vi "ConsolidateTerminals.vi"(1 "Terminal Set":T1(array[cluster])) -> (0 "Terminal Set":T1(array[cluster]))   [LabVIEW 2012, in "CThread.lvlib"]
uses:
  CThread.lvlib
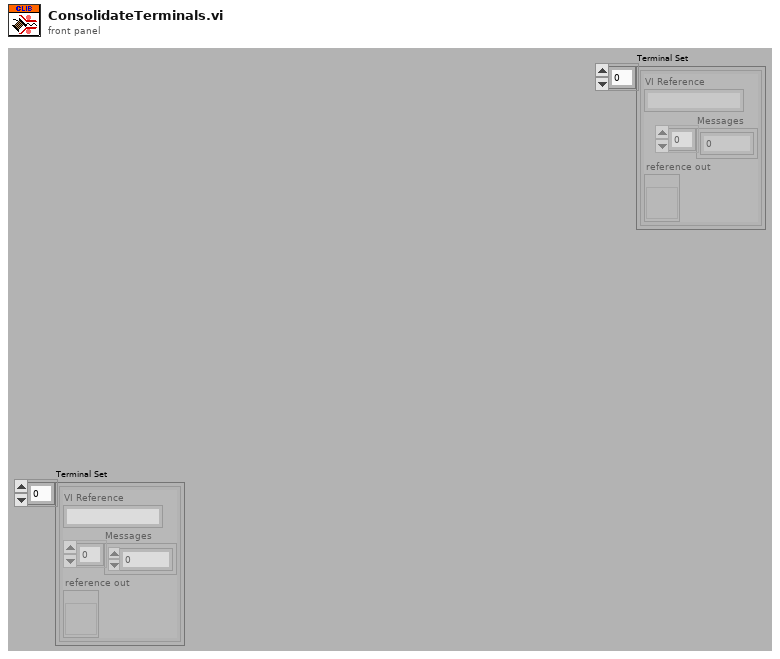
[diagram p1: front panel]
types:
  T1 = cluster{"VI Reference":string, "Messages":u8[], "reference out":refnum<vi>}[]
  T2 = cluster{"VI Reference":string, "Messages":u8[], "reference out":refnum<vi>}
  T3 = cluster{"VI Reference":string, "Combined Messages":u8[], "reference out":refnum<vi>}
  T4 = typedef "CRef.lvlib/Master Types.ctl" = enum8{"Null", "Boolean", "U8", "I8", "U16", "I16", "U32", "I32", "U64", "I64", "Single", "Double", "Extended", "CSG", "CDB", "CXT", "Boolean(Def)", "U8(Def)", "I8(Def)", "U16(Def)", "I16(Def)", "U32(Def)", "I32(Def)", "Reserved Def", "Reserved Def1", "Single(Def)", "Double(Def)", "Reserved Def2", "Reserved Def3", "Reserved Def4", "Reserved Def5", "Unsigned(Def)", "Signed(Def)", "Real(Def)", "Reserved Def6", "Numeric(Def)", "String"}
  T5 = typedef "LVRectTypeDef.ctl" = cluster{"Left":i16, "Top":i16, "Right":i16, "Bottom":i16}
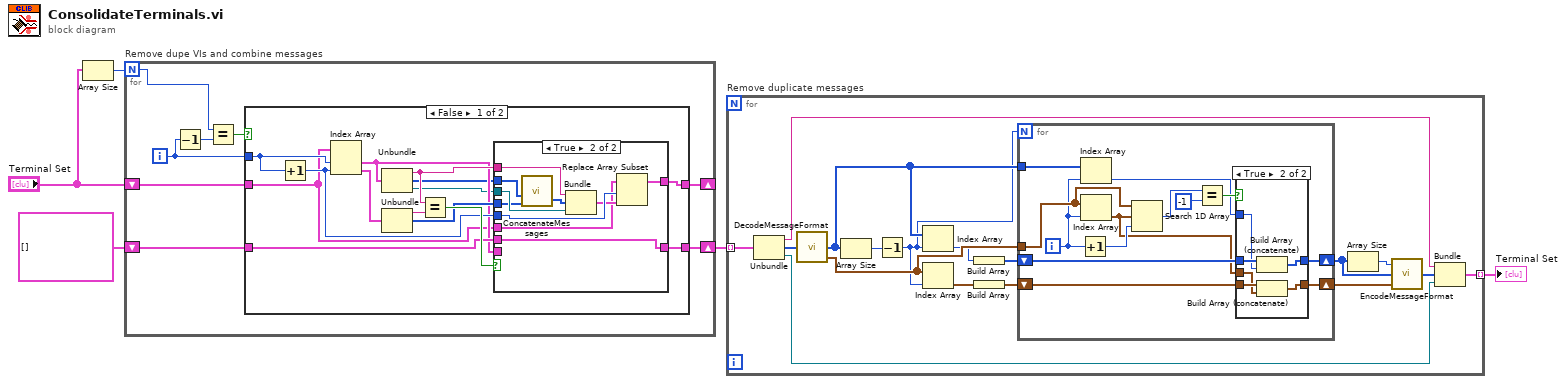
[diagram p0: block diagram]
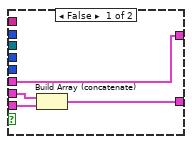
[diagram p3: hidden frame]
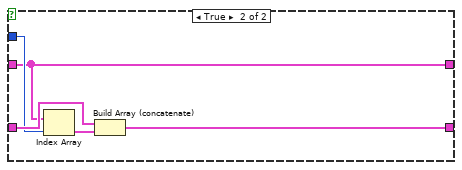
[diagram p4: hidden frame]
diagram:
  n1 = Array Size(array="Terminal Set") -> (size(s)=w5:i32)
  n2 = for "Remove dupe VIs and combine messages" {
    N: w5 -> [w13]
    shift-right: [w9] -> w2
    shift-left: T1 [] -> [w7]
    shift-right: [w6] -> _
    shift-left: "Terminal Set" -> [w8]
    i -> [w11]
    n3 = Decrement(x=w11) -> (x-1=w12:i32)
    n4 = Equal?(x=w13, y=w12) -> (x = y?=w10:bool)
    n5 = case shown="False" w10 {
      tunnel: w11 -> [w27 w44]
      tunnel: [w23 w46] -> w9
      tunnel: w8 -> [w17 w42]
      tunnel: w7 -> [w22 w45]
      tunnel: [w16 w42] -> w6
      frame False {
        n6 = Increment(x=w27) -> (x+1=w24:i32)
        n7 = Index Array(array=w17, index #1=w27, index #2=w24) -> (element #1=w18:T2, element #2=w26:T2)
        n8 = Unbundle(w18) -> ("VI Reference"=w19:string, "Messages"=w15:u8[], "reference out"=w14:refnum<vi>)
        n9 = Unbundle(w26) -> ("VI Reference"=w21:string, "Messages"=w20:u8[])  [unwired: 1 out]
        n10 = Equal?(x=w19, y=w21) -> (x = y?=w25:bool)
        n11 = case shown="True" w25 {
          tunnel: w24 -> [_ w41]
          tunnel: w22 -> [w31 w36]
          tunnel: [w30 w36] -> w23
          tunnel: w15 -> [_ w33]
          tunnel: w20 -> [_ w32]
          tunnel: w19 -> [_ w40]
          tunnel: w18 -> [w29 _]
          tunnel: w17 -> [w28 w38]
          tunnel: [w28 w37] -> w16
          tunnel: w14 -> [_ w35]
          frame False {
            n12 = Build Array (concatenate)(w31, w29) -> (w30:T1)
          }
          frame True {
            n13 = call "ConcatenateMessages.vi"("Messages 2"=w32, "Messages"=w33) -> ("Combined Messages"=w34:u8[])  [unwired: 3 in]
            n14 = Bundle("VI Reference"=w40, "Combined Messages"=w34, "reference out"=w35) -> (w39:T3)  [unwired: 1 in]
            n15 = Replace Array Subset(array=w38, new element=w39, index=w41) -> (w37:T1)
          }
        }
      }
      frame True {
        n16 = Index Array(array=w42, index=w44) -> (element=w43:T2)
        n17 = Build Array (concatenate)(w45, w43) -> (w46:T1)
      }
    }
  }
  n18 = for "Remove duplicate messages" {
    tunnel: w2 -> [w63] mode=indexing
    tunnel: [w57] -> w1 mode=indexing
    n19 = Unbundle(w63) -> ("VI Reference"=w60:string, "Messages"=w62:u8[], "reference out"=w59:refnum<vi>)
    n20 = call "DecodeMessageFormat.vi"("Messages"=w62) -> ("CRef Types"=w53:T4[], "Terminal Bounds[]"=w52:T5[])  [unwired: 2 in, 1 out]
    n21 = Array Size(array=w53) -> (size(s)=w56:i32)
    n22 = Decrement(x=w56) -> (x-1=w51:i32)
    n23 = Index Array(array=w53, index=w51) -> (element=w50:T4)
    n24 = Index Array(array=w52, index=w51) -> (element=w49:T5)
    n25 = Build Array(w50) -> (w47:T4[])
    n26 = Build Array(w49) -> (w48:T5[])
    n27 = for {
      N: w51 -> [_]
      tunnel: w53 -> [w65]
      tunnel: w52 -> [w76]
      shift-right: [w71] -> w55
      shift-left: w47 -> [w69]
      shift-right: [w70] -> w54
      shift-left: w48 -> [w68]
      i -> [w66]
      n28 = Increment(x=w66) -> (x+1=w73:i32)
      n29 = Index Array(array=w65, index=w66) -> (element=w64:T4)
      n30 = Index Array(array=w76, index=w66) -> (element=w67:T5)
      n31 = Search 1D Array(1D array=w76, element=w67, start index (0)=w73) -> (index of element=w75:i32)
      n32 = Equal?(x=w75, y=-1) -> (x = y?=w72:bool)
      n33 = case shown="True" w72 {
        tunnel: [w78 w84] -> w71
        tunnel: [w77 w83] -> w70
        tunnel: w69 -> [w78 w82]
        tunnel: w68 -> [w77 w81]
        tunnel: w67 -> [_ w80]
        tunnel: w64 -> [_ w79]
        frame False {
        }
        frame True {
          n34 = Build Array (concatenate)(w82, w79) -> (w84:T4[])
          n35 = Build Array (concatenate)(w81, w80) -> (w83:T5[])
        }
      }
    }
    n36 = Array Size(array=w55) -> (size(s)=w61:i32)
    n37 = call "EncodeMessageFormat.vi"("# of terminals"=w61, "CRef Types"=w55, "Terminal Bounds[]"=w54) -> ("Messages"=w58:u8[])  [unwired: 2 in]
    n38 = Bundle("VI Reference"=w60, "Messages"=w58, "reference out"=w59) -> (w57:T2)  [unwired: 1 in]
  }
  "Terminal Set" <- w1
